vi "test Is OD Entry_1.vi"(11 "Test Case In":refnum<class "test EDS.lvclass">) -> (0 "error out":errorcluster, 3 "Test Case Out":refnum<class "test EDS.lvclass">)   [LabVIEW 2024, in "test EDS.lvclass"]
uses:
  test EDS.lvclass
  C:/Program Files/National Instruments/LabVIEW 2024/vi.lib/Astemes/LUnit/Test Case.lvclass
  <vilib>/Astemes/LUnit/Test Case.lvclass/Test Case.ctl
  <vilib>/Astemes/LUnit/Append Fail Result.vi
  <vilib>/Astemes/LUnit/Append Pass Result.vi
  <vilib>/Astemes/LUnit/Run In UI.vi
  <vilib>/Utility/error.llb/Clear Errors.vi
  <vilib>/Astemes/LUnit/Test Case.lvclass
  Core/Section Name/Section Name.lvclass
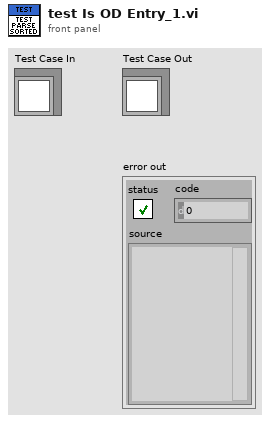
[diagram p1: front panel]
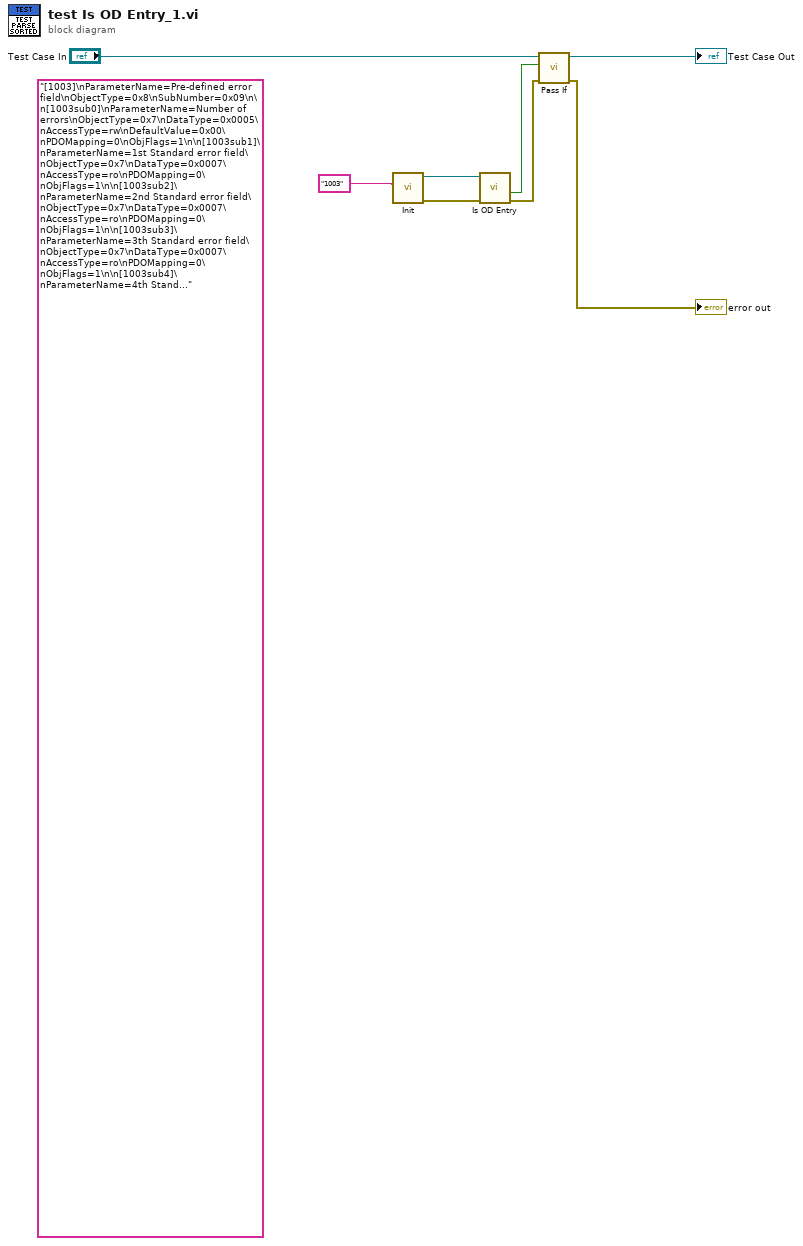
[diagram p0: block diagram]
diagram:
  (unwired) "[1003]\nParameterName=Pre-defined error field\nObjectType=0x8\nSubNumber=0x09\n\n[1003sub0]\nParameterName=Number of errors\nObjectType=0x7\nDataType=0x0005\nAccessType=rw\nDefaultValue=0x00\nPDOMapping=0\nObjFlags=1\n\n[1003sub1]\nParameterName=1st Standard error field\nObjectType=0x7\nDataType=0x0007\nAccessType=ro\nPDOMapping=0\nObjFlags=1\n\n[1003sub2]\nParameterName=2nd Standard error field\nObjectType=0x7\nDataType=0x0007\nAccessType=ro\nPDOMapping=0\nObjFlags=1\n\n[1003sub3]\nParameterName=3th Standard error field\nObjectType=0x7\nDataType=0x0007\nAccessType=ro\nPDOMapping=0\nObjFlags=1\n\n[1003sub4]\nParameterName=4th Standard error field\nObjectType=0x7\nDataType=0x0007\nAccessType=ro\nPDOMapping=0\nObjFlags=1\n\n[1003sub5]\nParameterName=5th Standard error field\nObjectType=0x7\nDataType=0x0007\nAccessType=ro\nPDOMapping=0\nObjFlags=1\n\n[1003sub6]\nParameterName=6th Standard error field\nObjectType=0x7\nDataType=0x0007\nAccessType=ro\nPDOMapping=0\nObjFlags=1\n\n[1003sub7]\nParameterName=7th Standard error field\nObjectType=0x7\nDataType=0x0007\nAccessType=ro\nPDOMapping=0\nObjFlags=1\n\n[1003sub8]\nParameterName=8th Standard error field\nObjectType=0x7\nDataType=0x0007\nAccessType=ro\nPDOMapping=0\nObjFlags=1"
  n1 = call "Init.vi"("Section Name"="1003") -> ("error out"=w4:errorcluster, "Section Name out"=w5:refnum<class "Section Name.lvclass">)  [unwired: 9 in]
  n2 = call "Is OD Entry.vi"("error in"=w4, "Section Name in"=w5) -> ("error out"=w2:errorcluster, "Is OD Entry?"=w1:bool)  [unwired: 6 in, 2 out]
  n3 = call <vilib>:"Pass If.vi"("error in (no error)"=w2, "Pass?"=w1, "LUnit Test Case In"="Test Case In") -> ("error out"=→"error out":errorcluster, "LUnit Test Case Out"=→"Test Case Out":refnum<class "test EDS.lvclass">)  [unwired: 7 in]
